vi "BoundsFinal.vi"(9 "N":dbl, 10 "Low":dbl, 11 "Hight":dbl) -> (0 "Res":dbl)   [LabVIEW 2023]
panel:
  out "tmp":dbl
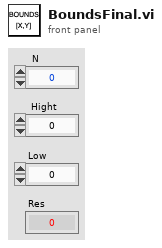
[diagram p1: front panel]
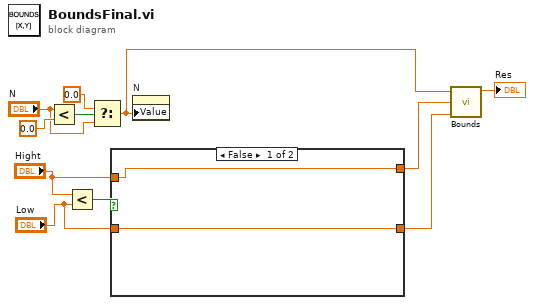
[diagram p0: block diagram]
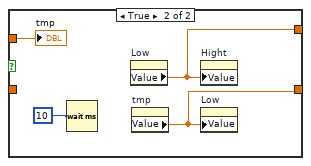
[diagram p2: hidden frame]
diagram:
  n1 = Less?(x="N", y=0.0) -> (x < y?=w10:bool)
  n2 = Less?(x="Hight", y="Low") -> (x < y?=w7:bool)
  n3 = Select(t=0.0, s=w10, f="N") -> (s? t:f=w5:dbl)
  n4 = case shown="False" w7 {
    tunnel: "Hight" -> [w13 w17]
    tunnel: [w13 w15] -> w4
    tunnel: [w12 w14] -> w3
    tunnel: "Low" -> [w12 _]
    frame False {
    }
    frame True {
      n5 = Wait (ms)(milliseconds to wait=u32 10) -> ()  [unwired: 1 out]
      n6 = property on="Low" class="DigNum (strict)"() -> ("Value"=w15:dbl)  [unwired: 2 in, 2 out]
      n7 = property on="tmp" class="DigNum (strict)"() -> ("Value"=w14:dbl)  [unwired: 2 in, 2 out]
      n8 = property on="Hight" class="DigNum (strict)"("Value"=w15) -> ()  [unwired: 2 in, 2 out]
      n9 = property on="Low" class="DigNum (strict)"("Value"=w14) -> ()  [unwired: 2 in, 2 out]
      "tmp" <- w17
    }
  }
  n10 = property on="N" class="DigNum (strict)"("Value"=w5) -> ()  [unwired: 2 in, 2 out]
  n11 = call "Bounds.vi"("Low"=w3, "Hight"=w4, "N"=w5) -> ("Res"=→"Res":dbl)  [unwired: 8 in]
